vi "sv_Swept Sine Gain and Phase.vi"(7 "reset":bool, 8 "unscaled measurements in":T1 {"harmonic components [ratio]" format="%.2f"; "THD [ratio]" format="%.2f"; "FRF Measurements"."Im [response]" format="%.2f"; "FRF Measurements"."Re [response]" format="%.2f"; "FRF Measurements"."Im [stimulus]" format="%.2f"; "FRF Measurements"."Re [stimulus]" format="%.2f"; "RMS response" format="%.2f"; "RMS stimulus" format="%.2f"}, 10 "frequency [normalized]":dbl format="%.2f", 11 "windowed data":cluster{"stimulus":dbl[], "response":dbl[]} {"response" format="%.2f"; "stimulus" format="%.2f"}) -> (0 "unscaled measurements out":T1 {"harmonic components [ratio]" format="%.2f"; "THD [ratio]" format="%.2f"; "FRF Measurements"."Im [response]" format="%.2f"; "FRF Measurements"."Re [response]" format="%.2f"; "FRF Measurements"."Im [stimulus]" format="%.2f"; "FRF Measurements"."Re [stimulus]" format="%.2f"; "RMS response" format="%.2f"; "RMS stimulus" format="%.2f"}, 3 "dup windowed data":cluster{"stimulus":dbl[], "response":dbl[]} {"response" format="%.2f"; "stimulus" format="%.2f"}, 5 "unscaled response magnitude":dbl format="%.3f")   [LabVIEW 2017, in "SoundVib_SweptSine.lvlib"]
uses:
  <vilib>/addons/Sound and Vibration/svt_Swept Sine/SoundVib_SweptSine.lvlib
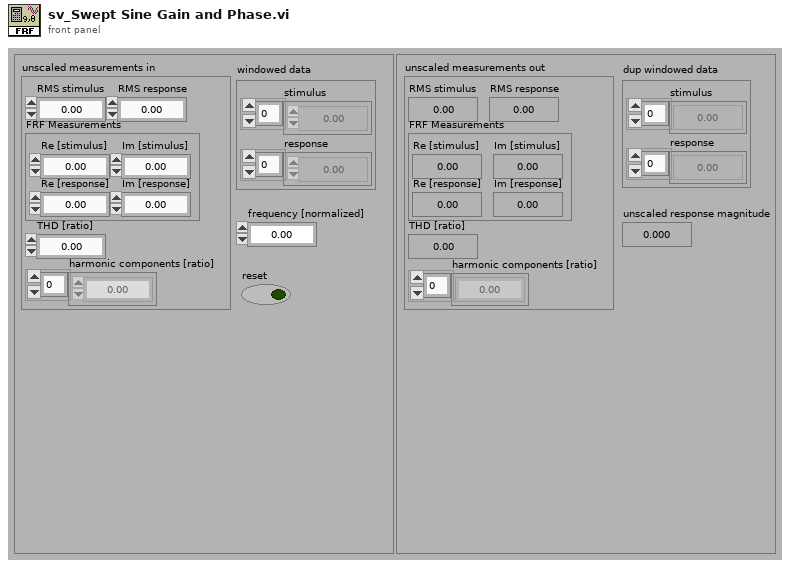
[diagram p1: front panel]
types:
  T1 = cluster{"RMS stimulus":dbl, "RMS response":dbl, "FRF Measurements":cluster{"Re [stimulus]":dbl, "Im [stimulus]":dbl, "Re [response]":dbl, "Im [response]":dbl}, "THD [ratio]":dbl, "harmonic components [ratio]":dbl[]}
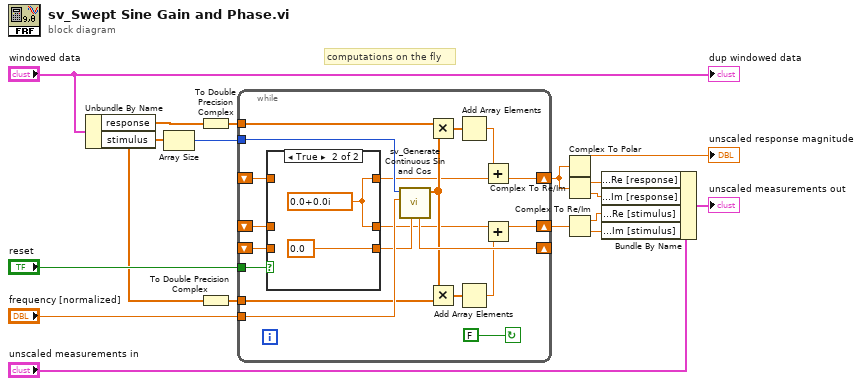
[diagram p0: block diagram]
diagram:
  # "computations on the fly"
  n1 = Unbundle By Name("windowed data") -> ("response"=w4:dbl[], "stimulus"=w2:dbl[])
  n2 = Array Size(array=w2) -> (size(s)=w16:i32)
  n3 = To Double Precision Complex(1:w4) -> (0:w3:cdb[])
  n4 = To Double Precision Complex(1:w2) -> (0:w1:cdb[])
  n5 = while {
    tunnel: w1 -> [w28]
    tunnel: w3 -> [w27]
    shift-right: [w29] -> w10
    shift-left: _ -> [w23]
    shift-right: [w30] -> w7
    shift-left: _ -> [w22]
    tunnel: "reset" -> [w26]
    tunnel: w16 -> [w32]
    tunnel: "frequency [normalized]" -> [w34]
    shift-right: [w33] -> _
    shift-left: _ -> [w24]
    stop <- FALSE continue-if-true
    # "final computations and export measurements"
    n6 = case shown="True" w26 {
      tunnel: [w40 0.0 ("sin phase in [degrees]")] -> w25
      tunnel: w24 -> [w40 _]
      tunnel: [w38 w41] -> w18
      tunnel: [w39 w41] -> w20
      tunnel: w23 -> [w39 _]
      tunnel: w22 -> [w38 _]
      frame False {
      }
      frame True {
        w41 = cdb 0.0+0.0i
      }
    }
    n7 = call <vilib>:"sv_Generate Continuous Sin and Cos.vi"("sin phase in [degrees]"=w25, "frequency [cycles/sample]"=w34, "number of samples"=w32) -> ("cos (theta) + i sin(theta)"=w31:cdb[], "sin phase out [degrees]"=w33:dbl)  [unwired: 7 in]
    n8 = Multiply(x=w27, y=w31) -> (x*y=w37:cdb[])
    n9 = Multiply(x=w31, y=w28) -> (x*y=w36:cdb[])
    n10 = Add Array Elements(numeric array=w37) -> (sum=w21:cdb)
    n11 = Add Array Elements(numeric array=w36) -> (sum=w19:cdb)
    n12 = Add(x=w21, y=w20) -> (x+y=w29:cdb)
    n13 = Add(x=w18, y=w19) -> (x+y=w30:cdb)
  }
  n14 = Complex To Polar(r * e^(i*theta)=w10) -> (r=→"unscaled response magnitude":dbl)  [unwired: 1 out]
  n15 = Complex To Re/Im(x + iy=w10) -> (x=w9:dbl, y=w8:dbl)
  n16 = Complex To Re/Im(x + iy=w7) -> (x=w6:dbl, y=w5:dbl)
  n17 = Bundle By Name(cluster="unscaled measurements in", "FRF Measurements.Re [response]"=w9, "FRF Measurements.Im [response]"=w8, "FRF Measurements.Re [stimulus]"=w6, "FRF Measurements.Im [stimulus]"=w5) -> (→"unscaled measurements out":T1)
  "dup windowed data" <- "windowed data"
